vi "Gyro.vi"() -> ()   [LabVIEW 2014]
uses:
  <vilib>/myRIO/Instrument Drivers/Onboard IO/I2C/typedefs/I2C User Configuration.ctl
  <vilib>/myRIO/Instrument Drivers/Onboard IO/I2C/typedefs/I2C Transfer Rate.ctl
  <vilib>/Platform/TimedLoop/XDataNode/timing_clust.ctl
  <vilib>/Platform/TimedLoop/XDataNode/nitl_modes.ctl
  <vilib>/Platform/TimedLoop/XDataNode/wakeup.ctl
  <vilib>/myRIO/Common/Instrument Driver Framework/myRIO v1.0/I2C/vis/myRIO v1.1 Open I2C.vi
  <vilib>/myRIO/Common/Instrument Driver Framework/Utilities/vis/Validate Channels.vi
  <vilib>/myRIO/Common/Instrument Driver Framework/myRIO v1.0/I2C/vis/myRIO v1.0 Reserve I2C.vi
  <vilib>/myRIO/Common/Instrument Driver Framework/myRIO v1.0/I2C/vis/myRIO v1.0 Build MUX Configuration I2C.vi
  <vilib>/myRIO/Common/Instrument Driver Framework/myRIO v1.0/Resource Manager/vis/myRIO v1.0 Reserve Channel List.vi
  <vilib>/myRIO/Common/Instrument Driver Framework/myRIO v1.0/Resource Manager/vis/myRIO v1.0 Create Configuration List.vi
  <vilib>/myRIO/Common/Instrument Driver Framework/myRIO v1.0/Resource Manager/vis/myRIO v1.0 Reserve Channel.vi
  <vilib>/myRIO/Common/Instrument Driver Framework/myRIO v1.0/Resource Manager/vis/myRIO v1.0 Unreserve Channel.vi
  <vilib>/myRIO/Common/Instrument Driver Framework/myRIO v1.0/Resource Manager/vis/myRIO v1.0 Build Mutex Name.vi
  <vilib>/Utility/VariantDataType/GetNumericInfo.vi
  <vilib>/Utility/error.llb/Error Cluster From Error Code.vi
  <vilib>/myRIO/Common/Instrument Driver Framework/myRIO v1.0/myRIO v1.1 Open.vi
  <vilib>/myRIO/Common/Instrument Driver Framework/Utilities/vis/IO Manager.vi
  <vilib>/myRIO/Common/Instrument Driver Framework/Utilities/vis/Configuration Manager.vi
  <vilib>/myRIO/Common/Instrument Driver Framework/myRIO v1.0/Resource Manager/vis/myRIO v1.0 Configure IO.vi
  <vilib>/myRIO/Common/Instrument Driver Framework/myRIO v1.0/myRIO v1.0 Close.vi
  <vilib>/myRIO/Common/Instrument Driver Framework/myRIO v1.0/I2C/vis/myRIO v1.0 Configure I2C.vi
  <vilib>/myRIO/Common/Instrument Driver Framework/myRIO v1.0/I2C/vis/myRIO v1.0 Write I2C.vi
  <vilib>/myRIO/Common/Instrument Driver Framework/myRIO v1.0/I2C/vis/myRIO v1.0 Read I2C.vi
  <vilib>/platform/TimedLoop/XDataNode/XDataNode.xnode
  <vilib>/myRIO/Instrument Drivers/Onboard IO/I2C/I2C.lvlib
  <vilib>/Platform/TimedLoop/XDataNode/XDNodeRunTimeDep.lvlib
  <vilib>/ptbypt/NI_PtbyPt.lvlib
panel:
  out "Z displacement":dbl format="%#_5g"
  out "Z":dbl format="%#_5g"
  out "Z-":dbl format="%#_5g"
  out "Z+":dbl format="%#_5g"
  out "Z- displacement":dbl format="%#_5g"
  in  "reset integrator":bool
  out "Z+ displacement":dbl format="%#_5g"
  out "Angular displacement [LSB]":T1(graph)
  out "Angular rate [LSB/sec]":cluster{i16, dbl, i16}(graph)
  in  "[ESC]":bool
  # "Gyroscope demo"
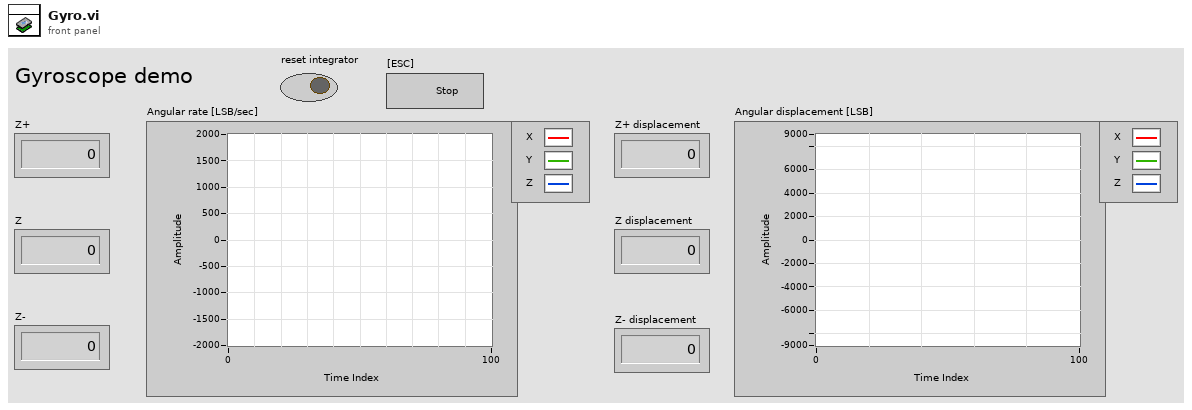
[diagram p1: front panel]
types:
  T1 = cluster{"integral x(t)":dbl, "integral x(t)":dbl, "integral x(t)":dbl}
  T2 = typedef "I2C.lvlib/I2C User Configuration.ctl" = cluster{"I2C Transfer Rate":T3}
  T3 = typedef "I2C.lvlib/I2C Transfer Rate.ctl" = enum16{"Standard mode (100 kbps)", "Fast mode (400 kbps)"}
  T4 = typedef "I2C.lvlib/I2C Reference.ctl" = cluster{"myRIO Reference":T5, "I2C Channels Enum":T9, "I2C Configuration":T10}
  T5 = typedef "myRIO Generic Hardware Reference.ctl" = cluster{"myRIO Model":T6, "myRIO Hardware Reference":T7}
  T6 = typedef "Hardware Version Enum.ctl" = enum16{"Unknown", "myRIO-1900", "myRIO-1950"}
  T7 = typedef "myRIO v1.0 Reference.ctl" = cluster{"Generic FPGA Reference":T8, "Allow multiple opens":bool}
  T8 = typedef "Generic FPGA Reference.ctl" = refnum<k20>
  T9 = typedef "I2C Channels Enum.ctl" = enum16{"Not Connected", "A/I2C", "B/I2C"}
  T10 = typedef "I2C.lvlib/I2C Configuration.ctl" = cluster{"I2C Transfer Rate":T3}
  T11 = typedef "XDNodeRunTimeDep.lvlib/timing_clust.ctl" = cluster{"Expected End [f-1]":u64, "Actual End [f-1]":u64, "Finished Late? [f-1]":bool, "Expected End [i-1]":u64, "Actual End [i-1]":u64, "Finished Late? [i-1]":bool, "Expected Start [i]":u64, "Actual Start [i]":u64, "Expected Start [f]":u64, "Actual Start [f]":u64, "Source Name":string, "Structure Name":string, "Period":i64, "Deadline":i64, "Offset":i64, "Start":i64, "Priority":i32, "Timeout":i32, "Mode":T12, "Wakeup Reason":T13, "Error":errorcluster, "Source Type":string, "Secondary Source Type":string, "Global End Time":u64, "Global Start Time":u64, "Frame Duration":u64, "Iteration Duration":u64, "Assigned CPU":i32, "I/O Scan Engine Mode":u32}
  T12 = typedef "XDNodeRunTimeDep.lvlib/nitl_modes.ctl" = enum32{"No Change", "Process missed periods, maintain original phase", "Discard missed periods, maintain original phase", "Process missed periods, ignore original phase", "Discard missed periods, ignore original phase"}
  T13 = typedef "XDNodeRunTimeDep.lvlib/wakeup.ctl" = enum32{"Normal", "Aborted", "Asynchronous wakeup", "Timing source error", "Timed loop error", "Timeout"}
  T14 = cluster{"integral x(t)":dbl, dbl, "integral x(t)":dbl}
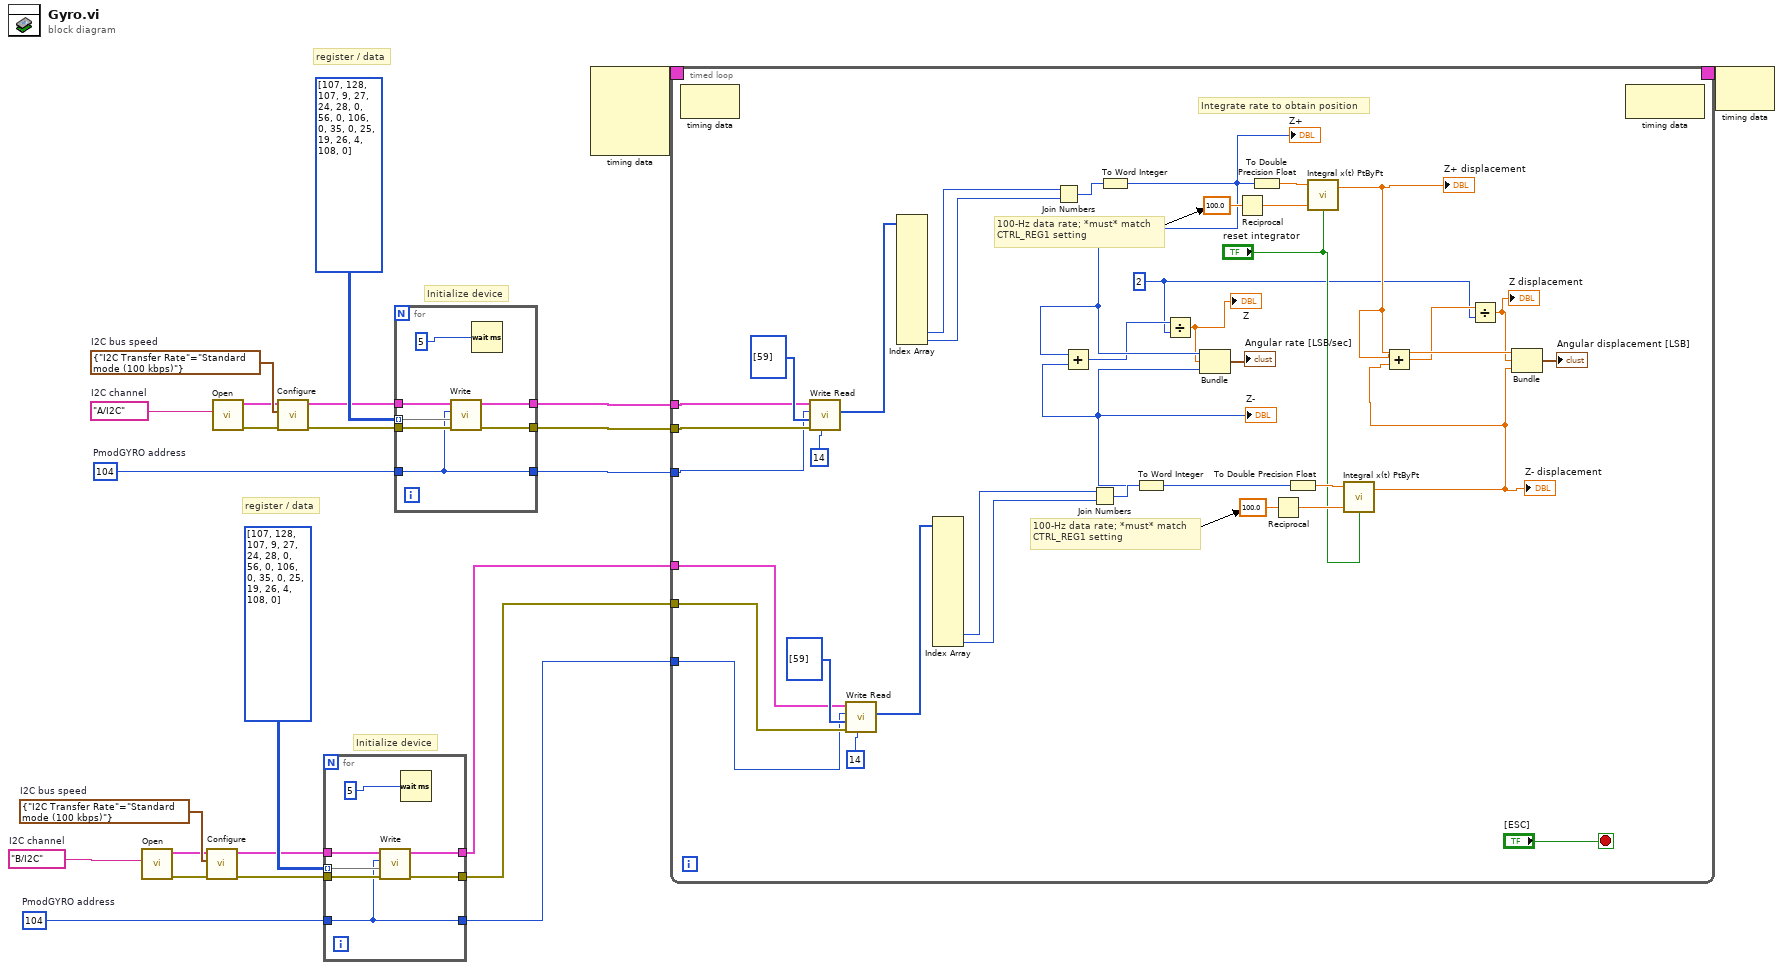
[diagram p0: block diagram]
diagram:
  w10 = T2 {"I2C Transfer Rate"=enum."Standard mode (100 kbps)"}  # I2C bus speed
  w11 = tag "B/I2C"  # I2C channel
  w4 = u8 104  # PmodGYRO address
  w23 = T2 {"I2C Transfer Rate"=enum."Standard mode (100 kbps)"}  # I2C bus speed
  w24 = tag "A/I2C"  # I2C channel
  w14 = u8 104  # PmodGYRO address
  # "Initialize device"
  # "register / data"
  # "Initialize device"
  # "register / data"
  n1 = call <vilib>:"Open.vi"("Channel Name"=w11) -> ("error out"=w8:errorcluster, "I2C Ref Out"=w9:T4)  [unwired: 9 in]
  n2 = call <vilib>:"Configure.vi"("error in (no error)"=w8, "I2C User Configuration"=w10, "I2C Ref In"=w9) -> ("error out"=w5:errorcluster, "I2C Ref Out"=w6:T4)  [unwired: 7 in]
  n3 = call <vilib>:"Open.vi"("Channel Name"=w24) -> ("error out"=w21:errorcluster, "I2C Ref Out"=w22:T4)  [unwired: 9 in]
  n4 = call <vilib>:"Configure.vi"("error in (no error)"=w21, "I2C User Configuration"=w23, "I2C Ref In"=w22) -> ("error out"=w15:errorcluster, "I2C Ref Out"=w16:T4)  [unwired: 7 in]
  n5 = for {
    tunnel: [w31] -> w2
    tunnel: [w30] -> w3
    tunnel: [w26] -> w1
    tunnel: u8[][] [[107, 128], [107, 9], [27, 24], [28, 0], [56, 0], [106, 0], [35, 0], [25, 19], [26, 4], [108, 0]] ("Bytes to Write") -> [w29] mode=indexing
    tunnel: w6 -> [w28]
    tunnel: w5 -> [w27]
    tunnel: w4 -> [w26]
    n6 = call <vilib>:"Write.vi"("error in (no error)"=w27, "Bytes to Write"=w29, "Slave Address (7-bit)"=w26, "I2C Ref In"=w28) -> ("error out"=w31:errorcluster, "I2C Ref Out"=w30:T4)  [unwired: 6 in]
    n7 = Wait (ms)(milliseconds to wait=5) -> ()  [unwired: 1 out]
  }
  n8 = for {
    tunnel: [w38] -> w20
    tunnel: [w37] -> w19
    tunnel: [w33] -> w18
    tunnel: u8[][] [[107, 128], [107, 9], [27, 24], [28, 0], [56, 0], [106, 0], [35, 0], [25, 19], [26, 4], [108, 0]] ("Bytes to Write") -> [w36] mode=indexing
    tunnel: w16 -> [w35]
    tunnel: w15 -> [w34]
    tunnel: w14 -> [w33]
    n9 = call <vilib>:"Write.vi"("error in (no error)"=w34, "Bytes to Write"=w36, "Slave Address (7-bit)"=w33, "I2C Ref In"=w35) -> ("error out"=w38:errorcluster, "I2C Ref Out"=w37:T4)  [unwired: 6 in]
    n10 = Wait (ms)(milliseconds to wait=5) -> ()  [unwired: 1 out]
  }
  n11 = node-c288() -> (w13:T11)  [unwired: 4 in]
  n12 = timed-loop {
    tunnel: w18 -> [w64]
    tunnel: w20 -> [w65]
    tunnel: w19 -> [w66]
    timing: w13 -> [_]
    timing-out: [_] -> w12
    tunnel: w3 -> [w51]
    tunnel: w2 -> [w50]
    tunnel: w1 -> [w49]
    stop <- "[ESC]" stop-if-true
    w39 = 2
    # "100-Hz data rate; *must* match\nCTRL_REG1 setting"
    # "100-Hz data rate; *must* match\nCTRL_REG1 setting"
    # "Integrate rate to obtain position"
    n13 = node-c288() -> ()  [unwired: 1 in, 1 out]
    n14 = call <vilib>:"Write Read.vi"("Byte Count"=u32 14, "error in (no error)"=w65, "Bytes to Write"=u8[] [59], "Slave Address (7-bit)"=w64, "I2C Ref In"=w66) -> ("Bytes Read"=w71:u8[])  [unwired: 3 in, 2 out]
    n15 = call <vilib>:"Write Read.vi"("Byte Count"=u32 14, "error in (no error)"=w50, "Bytes to Write"=u8[] [59], "Slave Address (7-bit)"=w49, "I2C Ref In"=w51) -> ("Bytes Read"=w57:u8[])  [unwired: 3 in, 2 out]
    n16 = Index Array "Index Array"(array=w71) -> (element #13=w62:u8, element #14=w61:u8)  [unwired: 14 in, 12 out]
    n17 = Index Array "Index Array"(array=w57) -> (element #13=w53:u8, element #14=w52:u8)  [unwired: 14 in, 12 out]
    n18 = Join Numbers(hi=w62, lo=w61) -> ((hi.lo)=w75:u16)
    n19 = Join Numbers(hi=w53, lo=w52) -> ((hi.lo)=w60:u16)
    n20 = To Word Integer(number=w75) -> (16bit integer=w47:i16)
    "Z+" <- w47
    n21 = To Word Integer(number=w60) -> (16bit integer=w46:i16)
    "Z-" <- w46
    n22 = Add(x=w47, y=w46) -> (x+y=w42:i16)
    n23 = Divide(x=w42, y=w39) -> (x/y=w43:dbl)
    "Z" <- w43
    n24 = Bundle "Bundle"(w47, w43, w46) -> (→"Angular rate [LSB/sec]":cluster{i16, dbl, i16})  [unwired: 1 in]
    n25 = Reciprocal(x=100.0 ("dt")) -> (1/x=w67:dbl)
    n26 = To Double Precision Float(number=w47) -> (double precision float=w70:dbl)
    n27 = Reciprocal(x=100.0 ("dt")) -> (1/x=w54:dbl)
    n28 = To Double Precision Float(number=w46) -> (double precision float=w56:dbl)
    n29 = call <vilib>:"Integral x(t) PtByPt.vi"("initialize"="reset integrator", "dt"=w67, "x"=w70) -> ("integral x(t)"=w45:dbl)  [unwired: 1 in, 1 out]
    "Z+ displacement" <- w45
    n30 = call <vilib>:"Integral x(t) PtByPt.vi"("initialize"="reset integrator", "dt"=w54, "x"=w56) -> ("integral x(t)"=w44:dbl)  [unwired: 1 in, 1 out]
    "Z- displacement" <- w44
    n31 = Add(x=w45, y=w44) -> (x+y=w40:dbl)
    n32 = Divide(x=w40, y=w39) -> (x/y=w41:dbl)
    "Z displacement" <- w41
    n33 = Bundle "Bundle"("integral x(t)"=w45, w41, "integral x(t)"=w44) -> (→"Angular displacement [LSB]":T14)  [unwired: 1 in]
    n34 = node-c288() -> ()  [unwired: 1 in, 1 out]
  }
  n35 = node-c288(w12) -> ()  [unwired: 1 out]
